vi "host.vi"() -> ()   [LabVIEW 2013]
uses:
  <vilib>/userdefined/High Color/nirio_resource_hc.ctl
  <instrlib>/niDCPower/nidcpower.llb/niDCPower Measurement Type.ctl
  <vilib>/FPGAPlugInAG/PXI-7953R/niLvFpga_Open_PXI-7953R.vi
  <vilib>/rvi/interface/common/dynamic/niFpgaDynamicAddResources.vi
  <vilib>/FPGAPlugInAG/Dynamic/niLvFpga_Reset_Dynamic.vi
  <vilib>/FPGAPlugInAG/Dynamic/niLvFpga_Run_Dynamic.vi
  <vilib>/rvi/interface/common/niFpgaWaitOnOcc.vi
  <vilib>/Utility/error.llb/Error Cluster From Error Code.vi
  <vilib>/rvi/errors/niLvFpgaAdjustHostInterfaceError.vi
  <vilib>/FPGAPlugInAG/Dynamic/niLvFpga_Close_Dynamic.vi
  <vilib>/rvi/interface/nirviOpenFPGA/nirviOpenFPGA.xnode
  FPGA Bitfiles/matrix_FPGATarget_Matrixtarget_8M6uhoGy8lc.lvbitx
  <vilib>/rvi/interface/nirviMethod/nirviMethod.xnode
  <vilib>/rvi/interface/nirviReadWriteControl/nirviReadWriteControl.xnode
  <vilib>/rvi/interface/nirviCloseFPGA/nirviCloseFPGA.xnode
  <vilib>/FPGAPlugInAG/Dynamic/niLvFpga_ReadFifo_Dynamic.vi
  <vilib>/rvi/errors/niLvFpgaMergeErrorWithErrorCode.vi
  <vilib>/rvi/interface/Simulation/niFpgaSimulationCallBeginRW.vi
  <vilib>/vision/NI_Vision_Development_Module.lvlib
  NiFpgaLv.dll
panel:
  in  "Мертвое время. мс":u32=200
  out "VAA_current, mA":dbl(graph)=0.09647506155015279
  out "VDDIO_current, mA":dbl(graph)=0.0007908422810211043
  out "VDD_current, mA":dbl(graph)=0.0007386855135800563
  in  "DELAY_i2c":u32=12
  out "Сумма сбоев":i32
  in  "Сброс Регистров":bool=TRUE
  out "Glitch Report":string
  in  "SEAL":bool
  in  "GLITCH":path=path "C:/TIM/Project/Matrix/Logs/Control/GLITCH"
  out "GLITCH_log file":refnum<file>
  in  "Index - Registers Page 2":u16[](array[numeric])=[2, 3, 4, 9, 10, 11, 12, 13, 14, 15, 16, 17, 65535, 65535, 65535, 21, 22, 23, 24, 25, 26, 27, 28, 29, 30, 31, 32, 33, 34, 35, 36, 38, 39, 40, 41, 42, 43, 44, 45, 46, 47, 65535, 65535, 65535, 51, 54, 55, 56, 57, 58, 59, 60, 61, 62, 65535, 70, 65535, 65535, 65535, 65535, 87, 88, 89, 90, 65535, 92, 93, 94, 95, 96, 65535, 65535, 65535, 100, 101, 103, 104, 130, 131, 132, 133, 134, 135, 136, 137, 138, 139, 140, 141, 142, 143, 144, 145, 146, 147, 148, 149, 150, 152, 153, 156, 180, 198, 200, 203, 204, 205, 206, 207, 208, 209, 210, 211, 212, 213, 239, 65535, 242, 65535, 244, 246, 247, 248, 249, 250, 251, 252, 253, 254, 255, 65535, 65535, 65535, 65535, 65535, 65535, 65535, 65535, 65534, 65535, 65535, 65531, 241, 242, 243, 244, 245, 246, 247, 248, 249, 250, 251, 252, 253, 254, 255]
  in  "Registers Page 2":u16[](array[numeric])=[110, 10531, 1316, 146, 22, 8, 171, 147, 88, 77, 169, 160, 65535, 65535, 65535, 373, 22, 67, 12, 0, 21, 31, 22, 152, 76, 160, 51220, 32896, 55648, 55648, 32512, 32768, 32776, 61188, 36211, 208, 24608, 24608, 61600, 3146, 57120, 65535, 65535, 65535, 5230, 30736, 768, 1088, 1676, 1676, 1676, 1676, 6105, 7423, 65535, 55552, 0, 65535, 65535, 65535, 537, 644, 537, 644, 2, 4620, 5394, 26684, 12296, 2, 32896, 65535, 65535, 23036, 0, 16400, 17, 1020, 769, 193, 929, 980, 983, 921, 1016, 28, 957, 987, 957, 1020, 990, 990, 990, 990, 31, 65, 867, 0, 255, 1, 57120, 32, 0, 0, 0, 0, 8608, 7835, 19018, 5773, 77, 0, 0, 520, 0, 8, 0, 0, 0, 110, 54, 13, 171, 136, 72, 87, 94, 122, 20543, 43136] format="%x"
  in  "current limit VDDIO":dbl=0.1 format="%#_13g"
  in  "voltage level VDDIO":dbl=2.5 format="%#_13g"
  in  "57":i16=57
  in  "91":i16=91
  in  "Index - Registers Page 1":u16[](array[numeric])=[5, 6, 8, 16, 17, 18, 27, 28, 30, 37, 52, 53, 58, 59, 60, 71, 72, 76, 77, 78, 82, 83, 84, 85, 86, 87, 88, 104, 128, 129, 130, 131, 132, 133, 134, 135, 136, 137, 138, 139, 140, 141, 142, 143, 144, 145, 146, 147, 148, 149, 155, 157, 159, 160, 161, 162, 163, 164, 165, 166, 167, 168, 169, 170, 174, 175, 179, 180, 181, 182, 183, 184, 185, 186, 187, 188, 189, 190, 191, 192, 193, 194, 195, 196, 200, 220, 221, 222, 223, 224, 225, 226, 227, 240]
  in  "Registers Page 1":u16[](array[numeric])=[3, 28686, 128, 61437, 64831, 16367, 0, 0, 512, 5, 16, 61456, 768, 1066, 1024, 24, 0, 0, 0, 10, 0, 7700, 17966, 34666, 47008, 57548, 0, 17, 7, 56588, 62696, 1276, 57868, 63212, 764, 56588, 62696, 250, 34866, 56754, 63466, 2, 47646, 60627, 63473, 255, 48926, 61142, 63474, 3, 512, 9390, 0, 1280, 1280, 0, 1024, 1024, 0, 1280, 640, 0, 1024, 512, 1284, 16, 2, 32, 257, 4363, 15399, 4362, 12834, 5643, 12836, 9228, 24124, 127, 8200, 20023, 100, 8463, 19250, 100, 0, 7700, 17966, 34666, 47008, 57548, 0, 28672, 45091, 0] format="%x"
  out "Glitch Registers":string
  out "glitch_num":i32
  out "Data_Read":u16 format="%x"
  in  "Index - Registers Page 0":u16[](array[numeric])=[0, 1, 2, 3, 4, 5, 6, 7, 8, 65535, 10, 11, 12, 13, 31, 32, 33, 34, 35, 36, 65535, 65535, 65535, 65535, 65535, 48, 49, 50, 51, 52, 54, 55, 65535, 60, 61, 65535, 63, 64, 65535, 66, 89, 90, 95, 96, 65535, 65535, 65535, 65535, 101, 112, 113, 114, 115, 116, 117, 118, 119, 120, 121, 122, 123, 124, 125, 126, 128, 129, 130, 131, 132, 133, 134, 135, 200, 240, 245, 246, 247, 248, 65535, 250, 251, 252, 253, 255, 65535]
  in  "Registers Page 0":u16[](array[numeric])=[5178, 12, 30, 1024, 487, 388, 42, 190, 17, 537, 17, 0, 0, 8, 0, 768, 1036, 297, 1544, 32875, 32, 32, 32, 32, 32, 1066, 7168, 0, 841, 49177, 61680, 0, 33, 6688, 8222, 8224, 8224, 8220, 215, 1911, 12, 49167, 8989, 128, 0, 0, 0, 0, 0, 31498, 31498, 6414, 6159, 22322, 22068, 29493, 12306, 30978, 29958, 30474, 30729, 32006, 12560, 126, 127, 127, 22282, 22539, 18188, 18446, 23298, 92, 0, 0, 2047, 2047, 0, 0, 124, 0, 0, 0, 0, 5178] format="%x"
  out "number":u64 format="%b"
  in  "WRITE\nSEL_LOG":bool=TRUE caption="SEL"
  out "SEL_log file":refnum<file>
  out "IS_SEL":bool
  in  "SIM_SEL":bool
  in  "VDDIO_limit, mA":dbl=20.0 format="%#_13g"
  in  "VAA_limit, mA":dbl=30.0 format="%#_13g"
  out "selNumVAA":i32 caption="selNum"
  out "selNumVDDIO":i32=3 caption="selNum"
  in  "voltage level VAA":dbl=2.8 format="%#_13g"
  in  "voltage level VDD":dbl=2.8 format="%#_13g"
  in  "current limit VAA":dbl=0.10000000000000009 format="%#_13g"
  in  "current limit VDD":dbl=0.1 format="%#_13g"
  in  "SEL":path=path "C:/TIM/Project/Matrix/Logs/Control/SEL"
  out "Температура":string="25"
  out "Номер образца":string="1"
  out "VDDIO_Current, mA":dbl=0.0007908422810211043 caption="mA" format="%_2g"
  out "VDDIO_Voltage, V":dbl=0.47498898751465163 caption="V" format="%_3g"
  out "VAA_Current, mA":dbl=0.09647506155015279 caption="mA" format="%_2g"
  out "VAA_Voltage, V":dbl=-0.00011092611436048789 caption="V" format="%_3g"
  in  "VAA - VAAPIX":refnum<k15>="PXI2Slot2"
  in  "SEL_time":u32=100
  out "Read_Low":u8 format="%x"
  out "Read_Up":u8 format="%x"
  out "TIRISTOR":bool
  in  "/RESET":bool=TRUE
  in  "DataLow":u8 format="%x"
  in  "Reg":u8=2 format="%x"
  in  "DataUp":u8 format="%x"
  in  "Device":u8=186 format="%x"
  in  "VDD_limit, mA":dbl=5.0 format="%#_13g"
  out "selNumVDD":i32 caption="selNum"
  out "Ready":bool
  in  "output enabled":bool
  out "VDD_Current, mA":dbl=0.0007386855135800563 caption="mA" format="%_2g"
  out "VDD_Voltage, V":dbl=0.00010885282841533817 caption="V" format="%_3g"
  in  "VDDIO - VDD":refnum<k15>="PXI2Slot3"
  in  "Comand":T1(ring)=enum."RGB565"
  in  "Height_pix":i32=250
  in  "Width_pix":i32=250
  in  "55":i16=55
  in  "73":i16=73
  in  "75":i16=75
  in  "56":i16=56
  in  "55":i16=55
  in  "Comand":bool
  out "ACK":u8 format="%b"
  out "String_counter":i16=250
  in  "String_number":i16=250
  in  "I2C_Request":bool
  in  "FALSE_LV":bool
  in  "FALSE_PIXCLK":bool
  in  "TRUE_FV":bool=TRUE
  in  "1_EXTCLK_divider":i16=3
  out "Image":T2(plugin-control)
  in  "0_WE divider":i32
  in  "50_Rise/Fall divider":i32=50
  in  "72":i16=72
  in  "18":i16=18
  in  "36":i16=36
  in  "54":i16=54
  in  "71":i16=71
  in  "17":i16=17
  in  "35":i16=35
  in  "53":i16=53
  in  "75_Stop":i16=75
  in  "100_Sclk_divider":i32=100
  in  "Read1":u8=255 format="%x"
  in  "Read2":u8=255 format="%x"
  in  "I2C_Write":bool=TRUE
  in  "stop":bool
  out "ArrayUp":u64=1408
  out "ArrayLow":u64=35465957116110822
  in  "resource name":T3="PXI2Slot6" caption="RIO Device"
  out "Сколько вначале":u32=125000
  out "Data":u8[](array[numeric])
  # "YCbCr mode"
  # "RGB565"
  # "LOGI"
  # "VDD"
  # "VDDIO"
  # "VAA"
  # "I2C"
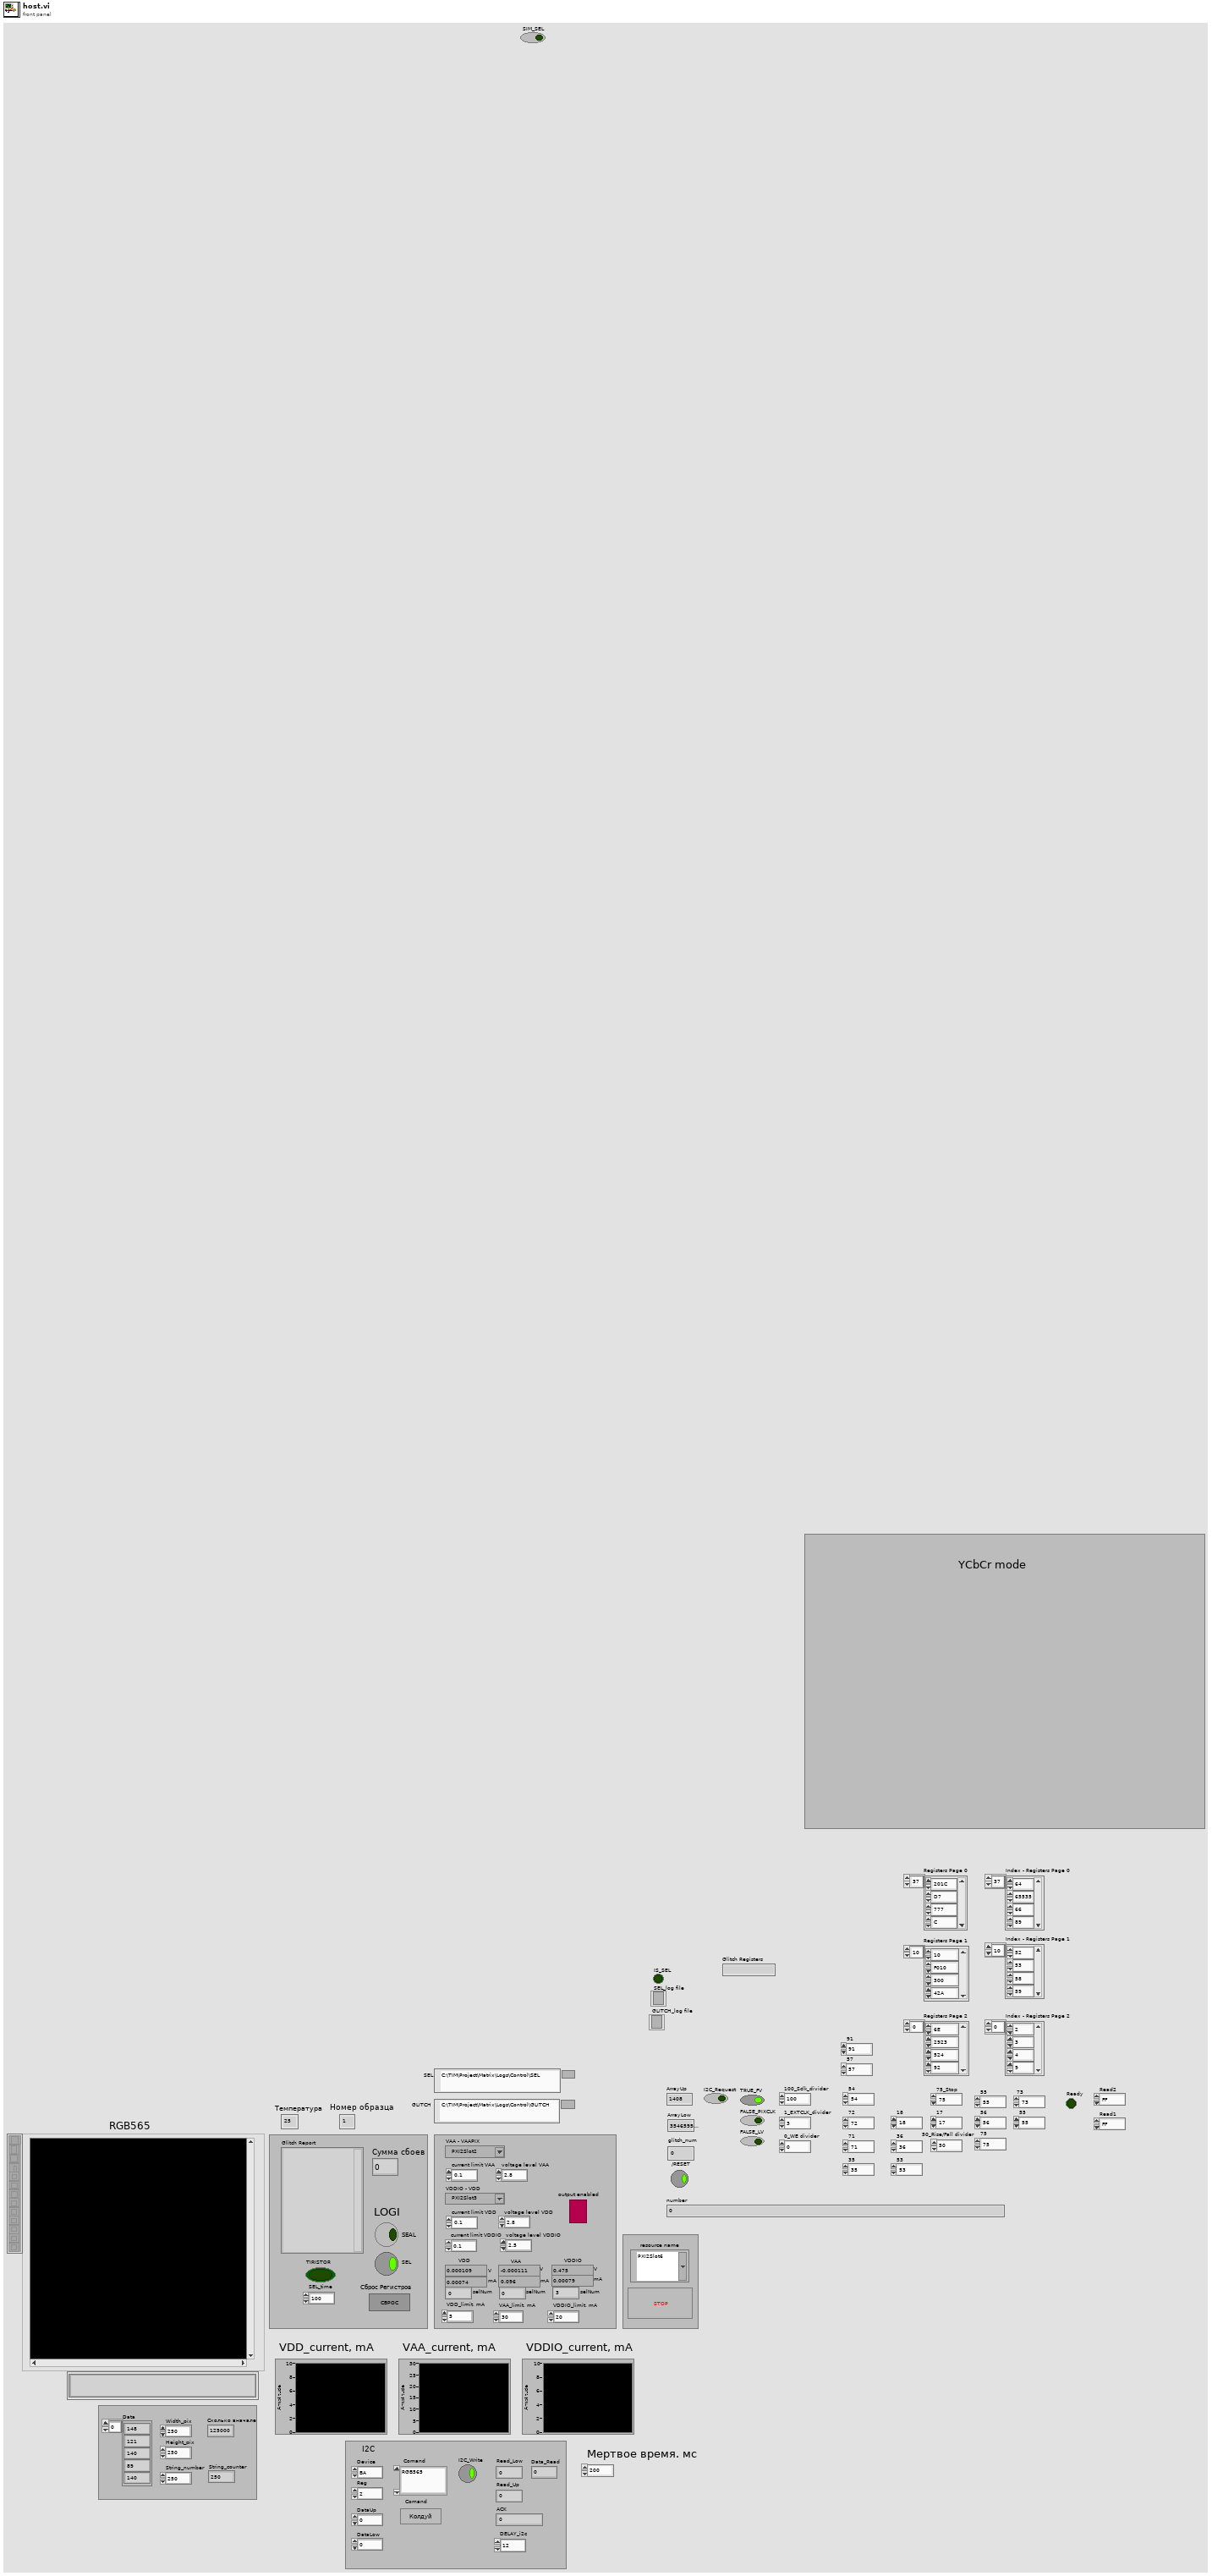
[diagram p1: front panel]
types:
  T1 = enum16{"check_registers", "From Controls", "250x250", "RGB565"}
  T2 = typedef "IMAQ Image.ctl" = refnum<image>
  T3 = typedef "nirio_resource_hc.ctl" = tag
  T4 = enum16{"open", "replace", "create", "open or create", "replace or create", "replace or create with confirmation"}
  T5 = typedef "niDCPower Measurement Type.ctl" = i32
  T6 = typedef "Image Type" = u32
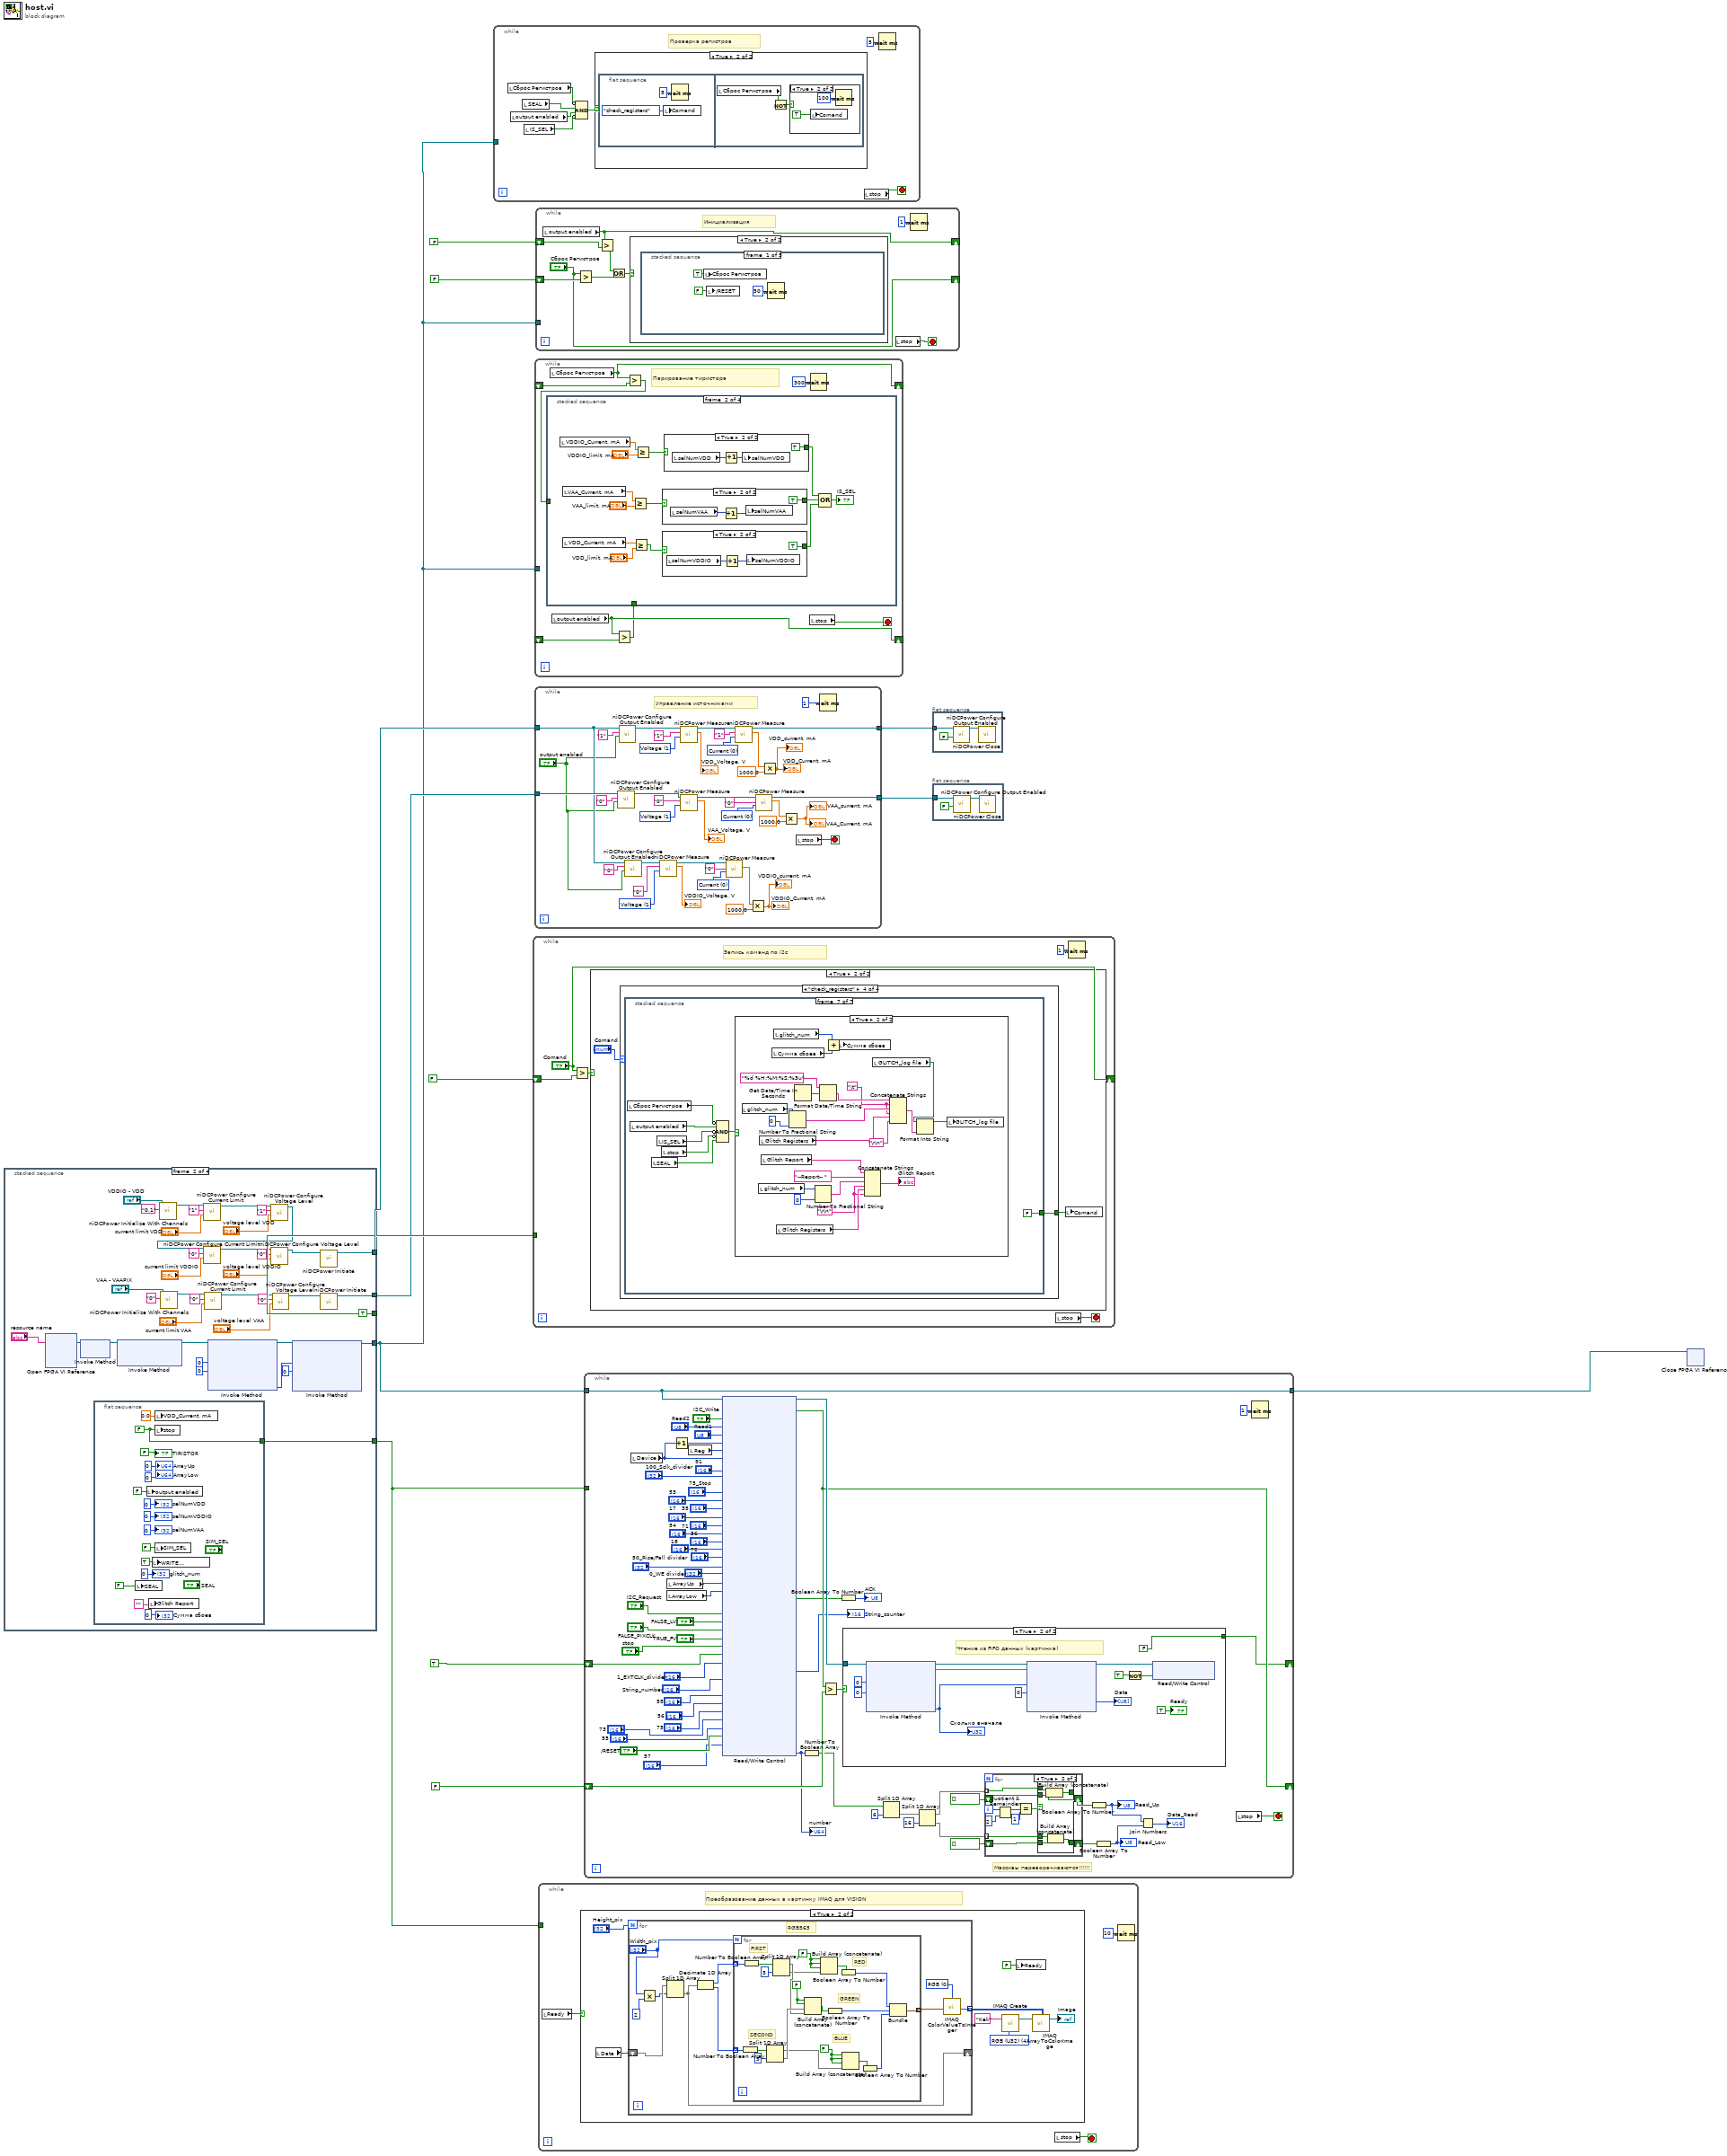
[diagram p0: block diagram]
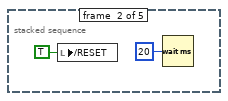
[diagram p3: hidden frame]
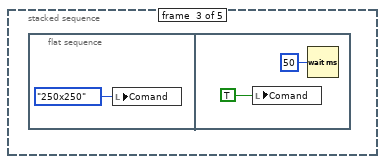
[diagram p4: hidden frame]
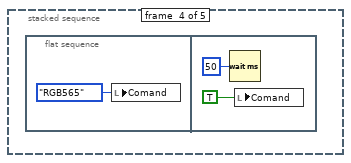
[diagram p5: hidden frame]
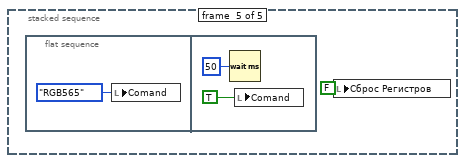
[diagram p6: hidden frame]
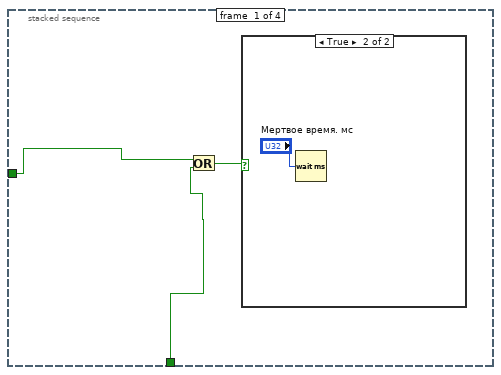
[diagram p10: hidden frame]
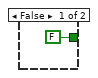
[diagram p12: hidden frame]
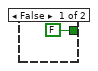
[diagram p13: hidden frame]
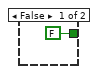
[diagram p14: hidden frame]
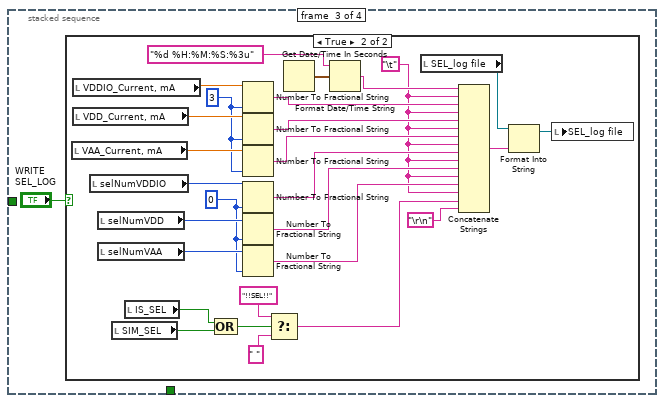
[diagram p15: hidden frame]
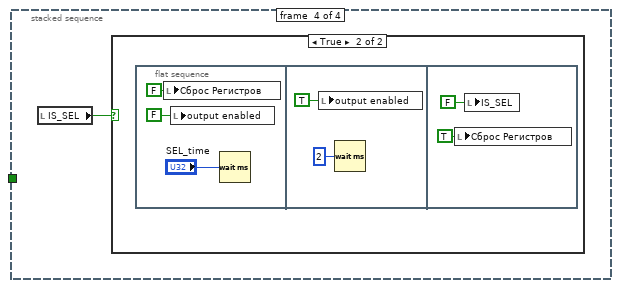
[diagram p17: hidden frame]
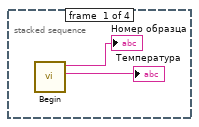
[diagram p19: hidden frame]
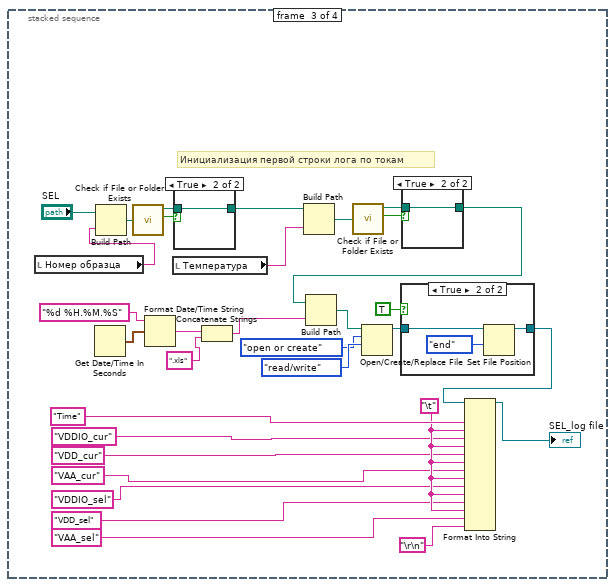
[diagram p20: hidden frame]
diagram:
  n1 = stacked-sequence {
    tunnel: [_ w53 _ _] -> w3
    tunnel: [_ w35 _ _] -> w6
    tunnel: [_ w34 _ _] -> w8
    tunnel: [_ TRUE _ _] -> w7
    tunnel: [_ w23 _ _] -> w5
    frame #0 {
      n2 = call "Begin.vi"() -> ("Температура 2"=→"Температура":string, "Номер образца 2"=→"Номер образца":string)  [unwired: 10 in]
    }
    frame #1 {
      n3 = xnode "Open FPGA VI Reference"("resource name"="resource name") -> ("FPGA VI Reference Out"=w44:refnum<k20>)  [unwired: 1 in, 1 out]
      n4 = xnode "Invoke Method"("FPGA VI Reference In"=w44) -> ("FPGA VI Reference Out"=w43:refnum<k20>)  [unwired: 1 in, 1 out]
      n5 = flat-sequence {
        tunnel: [w68] -> w35
        frame #0 {
          w68 = FALSE ("СТОП ПЛИС")
          n6 = local write "SEAL"(FALSE ("REGISTERS")) -> ()
          n7 = local write "output enabled"(FALSE ("output enabled")) -> ()
          n8 = local write "Glitch Report"("") -> ()
          n9 = local write "WRITE\nSEL_LOG"(TRUE ("WRITE\nSEL_LOG")) -> ()
          n10 = local write "VDD_Current, mA"(0.0 ("Ch1_Current, mA")) -> ()
          n11 = local write "stop"(w68) -> ()
          n12 = local write "SIM_SEL"(FALSE ("SIM_SEL")) -> ()
          "ArrayLow" <- u64 0 ("ArrayLow")
          "ArrayUp" <- u64 0 ("ArrayUp")
          "selNumVDD" <- 0 ("Numeric")
          "TIRISTOR" <- FALSE ("TIRISTOR")
          "selNumVDDIO" <- 0 ("Numeric")
          "selNumVAA" <- 0 ("Numeric")
          "glitch_num" <- 0 ("glitch_num")
          "Сумма сбоев" <- 0 ("glitch_sum")
        }
      }
      n13 = xnode "Invoke Method"("FPGA VI Reference In"=w43) -> ("FPGA VI Reference Out"=w41:refnum<k20>)  [unwired: 2 in, 1 out]
      n14 = call <instrlib>:"niDCPower Initialize With Channels.vi"("channels"="0,1", "resource name"="VDDIO - VDD") -> ("instrument handle out"=w45:refnum<k15>)  [unwired: 8 in, 1 out]
      n15 = call <instrlib>:"niDCPower Initialize With Channels.vi"("channels"="0", "resource name"="VAA - VAAPIX") -> ("instrument handle out"=w24:refnum<k15>)  [unwired: 8 in, 1 out]
      n16 = call <instrlib>:"niDCPower Configure Current Limit.vi"("current limit"="current limit VDD", "channel name"="1", "instrument handle"=w45) -> ("instrument handle out"=w46:refnum<k15>)  [unwired: 7 in, 1 out]
      n17 = call <instrlib>:"niDCPower Configure Current Limit.vi"("current limit"="current limit VAA", "channel name"="0", "instrument handle"=w24) -> ("instrument handle out"=w25:refnum<k15>)  [unwired: 7 in, 1 out]
      n18 = xnode "Invoke Method"("FPGA VI Reference In"=w41, "Number of Elements"=u32 0, "Timeout (ms)"=0) -> ("FPGA VI Reference Out"=w39:refnum<k20>, "Elements Remaining"=w40:u32)  [unwired: 1 in, 2 out]
      n19 = call <instrlib>:"niDCPower Configure Voltage Level.vi"("voltage level"="voltage level VDD", "channel name"="1", "instrument handle"=w46) -> ("instrument handle out"=w16:refnum<k15>)  [unwired: 7 in, 1 out]
      n20 = call <instrlib>:"niDCPower Configure Current Limit.vi"("current limit"="current limit VDDIO", "channel name"="0", "instrument handle"=w16) -> ("instrument handle out"=w22:refnum<k15>)  [unwired: 7 in, 1 out]
      n21 = call <instrlib>:"niDCPower Configure Voltage Level.vi"("voltage level"="voltage level VDDIO", "channel name"="0", "instrument handle"=w22) -> ("instrument handle out"=w17:refnum<k15>)  [unwired: 7 in, 1 out]
      n22 = call <instrlib>:"niDCPower Configure Voltage Level.vi"("voltage level"="voltage level VAA", "channel name"="0", "instrument handle"=w25) -> ("instrument handle out"=w26:refnum<k15>)  [unwired: 7 in, 1 out]
      n23 = xnode "Invoke Method"("FPGA VI Reference In"=w39, "Number of Elements"=w40, "Timeout (ms)"=0) -> ("FPGA VI Reference Out"=w53:refnum<k20>)  [unwired: 1 in, 3 out]
      n24 = call <instrlib>:"niDCPower Initiate.vi"("instrument handle"=w17) -> ("instrument handle out"=w34:refnum<k15>)  [unwired: 9 in, 1 out]
      n25 = call <instrlib>:"niDCPower Initiate.vi"("instrument handle"=w26) -> ("instrument handle out"=w23:refnum<k15>)  [unwired: 9 in, 1 out]
    }
    frame #2 {
      w77 = "\t"
      # "Инициализация первой строки лога по токам"
      n26 = local read "Номер образца"() -> (w88:string)
      n27 = Get Date/Time In Seconds() -> (seconds since 1Jan1904=w93:timestamp)
      n28 = Build Path(base path="SEL", name or relative path=w88) -> (appended path=w86:path)
      n29 = call <vilib>:"Check if File or Folder Exists.vi"("path"=w86) -> ("file or folder exists?"=w85:bool, "dup path"=w84:path)  [unwired: 8 in, 1 out]
      n30 = Format Date/Time String(time format string (%c)="%d %H.%M.%S", seconds (now)=w93) -> (date/time string=w95:string)  [unwired: 1 in]
      n31 = local read "Температура"() -> (w91:string)
      n32 = case shown="True" w85 {
        tunnel: w84 -> [w109 w110]
        tunnel: [w108 w110] -> w90
        frame False {
          n33 = Create Folder(path (use dialog)=w109) -> (created path=w108:path)  [unwired: 2 in, 2 out]
        }
        frame True {
        }
      }
      n34 = Concatenate Strings(w95, ".xls" ("string")) -> (w96:string)
      n35 = Build Path(base path=w90, name or relative path=w91) -> (appended path=w99:path)
      n36 = call <vilib>:"Check if File or Folder Exists.vi"("path"=w99) -> ("file or folder exists?"=w100:bool, "dup path"=w89:path)  [unwired: 8 in, 1 out]
      n37 = case shown="True" w100 {
        tunnel: w89 -> [w106 w107]
        tunnel: [w105 w107] -> w97
        frame False {
          n38 = Create Folder(path (use dialog)=w106) -> (created path=w105:path)  [unwired: 2 in, 2 out]
        }
        frame True {
        }
      }
      n39 = Build Path(base path=w97, name or relative path=w96) -> (appended path=w94:path)
      n40 = Open/Create/Replace File(file path (use dialog)=w94, operation (0:open)=T4."open or create", access (0:read/write)=enum16{"read/write", "read-only", "write-only"}."read/write") -> (refnum out=w92:refnum<file>)  [unwired: 3 in, 2 out]
      n41 = case shown="True" TRUE {
        tunnel: w92 -> [w101 w104]
        tunnel: [w101 w102] -> w98
        frame False {
        }
        frame True {
          n42 = Set File Position(refnum=w104, from (0:start)=enum16{"start", "end", "current"}."end") -> (refnum out=w102:refnum<file>)  [unwired: 2 in, 1 out]
        }
      }
      n43 = Format Into String(initial string=w98, "Time" ("input 1"), w77, "VDDIO_cur" ("input 1"), w77, "VDD_cur" ("input 1"), w77, "VAA_cur" ("input 1"), w77, "VDDIO_sel" ("input 1"), w77, "VDD_sel" ("input 1"), w77, "VAA_sel" ("input 1"), "\r\n") -> (resulting string=→"SEL_log file":refnum<file>)  [unwired: 2 in, 1 out]
    }
    frame #3 {
      w115 = "\t"
      # "Инициализация первой строки лога по сбоям"
      n44 = local read "Номер образца"() -> (w126:string)
      n45 = Get Date/Time In Seconds() -> (seconds since 1Jan1904=w131:timestamp)
      n46 = Build Path(base path="GLITCH", name or relative path=w126) -> (appended path=w124:path)
      n47 = call <vilib>:"Check if File or Folder Exists.vi"("path"=w124) -> ("file or folder exists?"=w123:bool, "dup path"=w122:path)  [unwired: 8 in, 1 out]
      n48 = Format Date/Time String(time format string (%c)="%d %H.%M.%S", seconds (now)=w131) -> (date/time string=w133:string)  [unwired: 1 in]
      n49 = local read "Температура"() -> (w129:string)
      n50 = case shown="True" w123 {
        tunnel: w122 -> [w147 w148]
        tunnel: [w146 w148] -> w128
        frame False {
          n51 = Create Folder(path (use dialog)=w147) -> (created path=w146:path)  [unwired: 2 in, 2 out]
        }
        frame True {
        }
      }
      n52 = Concatenate Strings(w133, ".xls" ("string")) -> (w134:string)
      n53 = Build Path(base path=w128, name or relative path=w129) -> (appended path=w137:path)
      n54 = call <vilib>:"Check if File or Folder Exists.vi"("path"=w137) -> ("file or folder exists?"=w138:bool, "dup path"=w127:path)  [unwired: 8 in, 1 out]
      n55 = case shown="True" w138 {
        tunnel: w127 -> [w144 w145]
        tunnel: [w143 w145] -> w135
        frame False {
          n56 = Create Folder(path (use dialog)=w144) -> (created path=w143:path)  [unwired: 2 in, 2 out]
        }
        frame True {
        }
      }
      n57 = Build Path(base path=w135, name or relative path=w134) -> (appended path=w132:path)
      n58 = Open/Create/Replace File(file path (use dialog)=w132, operation (0:open)=T4."open or create", access (0:read/write)=enum16{"read/write", "read-only", "write-only"}."read/write") -> (refnum out=w130:refnum<file>)  [unwired: 3 in, 2 out]
      n59 = case shown="True" TRUE {
        tunnel: w130 -> [w139 w142]
        tunnel: [w139 w140] -> w136
        frame False {
        }
        frame True {
          n60 = Set File Position(refnum=w142, from (0:start)=enum16{"start", "end", "current"}."end") -> (refnum out=w140:refnum<file>)  [unwired: 2 in, 1 out]
        }
      }
      n61 = Format Into String(initial string=w136, "Time" ("input 1"), w115, "Glitch Number" ("input 1"), w115, "Registers" ("input 1"), "\r\n") -> (resulting string=→"GLITCH_log file":refnum<file>)  [unwired: 2 in, 1 out]
    }
  }
  n62 = while {
    tunnel: w3 -> [_]
    stop <- w155 stop-if-true
    # "Проверка регистров"
    n63 = local read "Сброс Регистров"() -> (w149:bool)
    n64 = local read "output enabled"() -> (w153:bool)
    n65 = local read "SEAL"() -> (w152:bool)
    n66 = local read "IS_SEL"() -> (w151:bool)
    n67 = Compound Arithmetic op=AND(invert w149, w152, w153, invert w151) -> (w150:bool)
    n68 = case shown="True" w150 {
      frame False {
      }
      frame True {
        n69 = flat-sequence {
          frame #0 {
            n70 = local write "Comand"(T1."check_registers" ("Comand")) -> ()
            n71 = Wait (ms)(milliseconds to wait=u32 5) -> ()  [unwired: 1 out]
          }
          frame #1 {
            n72 = local read "Сброс Регистров"() -> (w159:bool)
            n73 = Not(x=w159) -> (.not. x?=w158:bool)
            n74 = case shown="True" w158 {
              frame False {
              }
              frame True {
                n75 = local write "Comand"(TRUE) -> ()
                n76 = Wait (ms)(milliseconds to wait=u32 100) -> ()  [unwired: 1 out]
              }
            }
          }
        }
      }
    }
    n77 = local read "stop"() -> (w155:bool)
    n78 = Wait (ms)(milliseconds to wait=u32 5) -> ()  [unwired: 1 out]
  }
  n79 = while {
    shift-right: ["Comand"] -> _
    shift-left: FALSE -> [w164]
    tunnel: w7 -> [_]
    stop <- w166 stop-if-true
    # "Запись команд по i2c"
    n80 = Greater?(x="Comand", y=w164) -> (0:w165:bool)
    n81 = case shown="True" w165 {
      frame False {
      }
      frame True {
        n82 = case shown="\"check_registers\"" "Comand" {
          tunnel: [w169 w195 w220 w232] -> w167
          frame "RGB565" {
            n83 = stacked-sequence {
              tunnel: [_ w181] -> w169
              frame #0 {
                n84 = flat-sequence {
                  frame #0 {
                    n85 = local write "I2C_Write"(TRUE ("I2C_Write")) -> ()
                    n86 = call "I2C_Write.vi"("DataLow"=u8 1 ("Device"), "DataUp"=u8 0 ("Device"), "Reg"=u8 240 ("Device"), "Device"=u8 186) -> ("ArrayLow"=w175:u64, "ArrayUp"=w174:u64)  [unwired: 6 in]
                    n87 = local write "ArrayUp"(w174) -> ()
                    n88 = local write "ArrayLow"(w175) -> ()
                  }
                  frame #1 {
                    n89 = local write "I2C_Request"(TRUE ("I2C_Request")) -> ()
                    n90 = Wait (ms)(milliseconds to wait=u32 20) -> ()  [unwired: 1 out]
                  }
                  frame #2 {
                    n91 = local write "I2C_Request"(FALSE ("I2C_Request")) -> ()
                    n92 = Wait (ms)(milliseconds to wait=u32 10) -> ()  [unwired: 1 out]
                  }
                }
              }
              frame #1 {
                n93 = flat-sequence {
                  tunnel: [FALSE ("RGB565")] -> w181
                  frame #0 {
                    n94 = local write "I2C_Write"(TRUE ("I2C_Write")) -> ()
                    n95 = call "I2C_Write.vi"("DataLow"=u8 0 ("Device"), "DataUp"=u8 3 ("Device"), "Reg"=u8 58 ("Device"), "Device"=u8 186) -> ("ArrayLow"=w187:u64, "ArrayUp"=w186:u64)  [unwired: 6 in]
                    n96 = local write "ArrayUp"(w186) -> ()
                    n97 = local write "ArrayLow"(w187) -> ()
                  }
                  frame #1 {
                    n98 = local write "I2C_Request"(TRUE ("I2C_Request")) -> ()
                    n99 = Wait (ms)(milliseconds to wait=u32 20) -> ()  [unwired: 1 out]
                  }
                  frame #2 {
                    n100 = local write "I2C_Request"(FALSE ("I2C_Request")) -> ()
                    n101 = Wait (ms)(milliseconds to wait=u32 10) -> ()  [unwired: 1 out]
                  }
                }
              }
            }
          }
          frame "250x250" {
            w194 = 250 ("Height_pix")
            n102 = stacked-sequence {
              tunnel: [_ w207] -> w195
              frame #0 {
                n103 = flat-sequence {
                  frame #0 {
                    n104 = local write "I2C_Write"(TRUE ("I2C_Write")) -> ()
                    n105 = call "I2C_Write.vi"("DataLow"=u8 0 ("Device"), "DataUp"=u8 0 ("Device"), "Reg"=u8 240 ("Device"), "Device"=u8 186) -> ("ArrayLow"=w201:u64, "ArrayUp"=w200:u64)  [unwired: 6 in]
                    n106 = local write "ArrayUp"(w200) -> ()
                    n107 = local write "ArrayLow"(w201) -> ()
                  }
                  frame #1 {
                    n108 = local write "I2C_Request"(TRUE ("I2C_Request")) -> ()
                    n109 = Wait (ms)(milliseconds to wait=u32 10) -> ()  [unwired: 1 out]
                  }
                  frame #2 {
                    n110 = local write "I2C_Request"(FALSE ("I2C_Request")) -> ()
                    n111 = Wait (ms)(milliseconds to wait=u32 10) -> ()  [unwired: 1 out]
                  }
                }
              }
              frame #1 {
                n112 = flat-sequence {
                  tunnel: [FALSE ("RGB565")] -> w207
                  frame #0 {
                    n113 = local write "I2C_Write"(TRUE ("I2C_Write")) -> ()
                    n114 = call "I2C_Write.vi"("DataLow"=u8 231 ("Device"), "DataUp"=u8 1 ("Device"), "Reg"=u8 4 ("Device"), "Device"=u8 186) -> ("ArrayLow"=w209:u64, "ArrayUp"=w208:u64)  [unwired: 6 in]
                    n115 = local write "ArrayUp"(w208) -> ()
                    n116 = local write "ArrayLow"(w209) -> ()
                  }
                  frame #1 {
                    n117 = local write "I2C_Request"(TRUE ("I2C_Request")) -> ()
                    n118 = Wait (ms)(milliseconds to wait=u32 10) -> ()  [unwired: 1 out]
                  }
                  frame #2 {
                    n119 = local write "I2C_Request"(FALSE ("I2C_Request")) -> ()
                    n120 = Wait (ms)(milliseconds to wait=u32 10) -> ()  [unwired: 1 out]
                  }
                }
              }
            }
            n121 = local write "String_number"(w194) -> ()
            n122 = local write "Width_pix"(w194) -> ()
            n123 = local write "Height_pix"(w194) -> ()
          }
          frame "From Controls" {
            n124 = flat-sequence {
              tunnel: [FALSE] -> w220
              frame #0 {
                n125 = call "I2C_Write.vi"("DataLow"="DataLow", "DataUp"="DataUp", "Reg"="Reg", "Device"="Device") -> ("ArrayLow"=w222:u64, "ArrayUp"=w221:u64)  [unwired: 6 in]
                n126 = local write "ArrayUp"(w221) -> ()
                n127 = local write "ArrayLow"(w222) -> ()
              }
              frame #1 {
                n128 = local write "I2C_Request"(TRUE ("I2C_Request")) -> ()
                n129 = Wait (ms)(milliseconds to wait=u32 20) -> ()  [unwired: 1 out]
              }
              frame #2 {
                n130 = local write "I2C_Request"(FALSE ("I2C_Request")) -> ()
                n131 = Wait (ms)(milliseconds to wait=u32 1) -> ()  [unwired: 1 out]
              }
            }
          }
          frame "check_registers" {
            n132 = stacked-sequence {
              tunnel: [_ _ _ _ _ _ FALSE ("RGB565")] -> w232
              frame #0 {
                n133 = flat-sequence {
                  frame #0 {
                    n134 = local write "I2C_Write"(TRUE ("I2C_Write")) -> ()
                    n135 = call "I2C_Write.vi"("DataLow"=u8 0 ("Device"), "DataUp"=u8 0 ("Device"), "Reg"=u8 240 ("Device"), "Device"=u8 186) -> ("ArrayLow"=w238:u64, "ArrayUp"=w237:u64)  [unwired: 6 in]
                    n136 = local write "ArrayUp"(w237) -> ()
                    n137 = local write "ArrayLow"(w238) -> ()
                  }
                  frame #1 {
                    n138 = local write "I2C_Request"(TRUE ("I2C_Request")) -> ()
                    n139 = Wait (ms)(milliseconds to wait="DELAY_i2c") -> ()  [unwired: 1 out]
                  }
                  frame #2 {
                    n140 = local write "I2C_Request"(FALSE ("I2C_Request")) -> ()
                    n141 = Wait (ms)(milliseconds to wait=u32 2) -> ()  [unwired: 1 out]
                  }
                }
              }
              frame #1 {
                # "PAGE 0"
                n142 = local write "glitch_num"(0 ("glitch_num")) -> ()
                n143 = local write "I2C_Write"(FALSE ("I2C_Write")) -> ()
                n144 = while {
                  tunnel: "Index - Registers Page 0" -> [w264] mode=indexing
                  tunnel: "Registers Page 0" -> [w263] mode=indexing
                  shift-right: [w261] -> w246
                  shift-left: "" -> [w262]
                  i -> [w257]
                  stop <- w255 stop-if-true
                  n145 = stacked-sequence {
                    tunnel: w264 -> [w266 _ w270]
                    tunnel: w263 -> [_ _ w275]
                    tunnel: w262 -> [_ _ w279]
                    tunnel: [_ _ w278] -> w261
                    frame #0 {
                      n146 = local write "Device"(u8 186 ("Device")) -> ()
                      n147 = local write "Reg"(w266) -> ()
                      n148 = Wait (ms)(milliseconds to wait=u32 4) -> ()  [unwired: 1 out]
                    }
                    frame #1 {
                      n149 = local write "I2C_Request"(TRUE ("I2C_Request")) -> ()
                      n150 = local read "DELAY_i2c"() -> (w268:u32)
                      n151 = Wait (ms)(milliseconds to wait=w268) -> ()  [unwired: 1 out]
                    }
                    frame #2 {
                      n152 = local read "Data_Read"() -> (w277:u16)
                      n153 = local write "I2C_Request"(FALSE ("I2C_Request")) -> ()
                      n154 = Equal?(x=w275, y=w277) -> (x = y?=w272:bool)
                      n155 = Equal?(x=w270, y=u16 65535) -> (x = y?=w274:bool)
                      n156 = Or(x=w272, y=w274) -> (x .or. y?=w271:bool)
                      n157 = case shown="False" w271 {
                        tunnel: w279 -> [w292 w295]
                        tunnel: [w291 w295] -> w278
                        tunnel: w270 -> [w289 _]
                        tunnel: w277 -> [w285 _]
                        tunnel: w275 -> [w281 _]
                        frame False {
                          n158 = local read "glitch_num"() -> (w294:i32)
                          n159 = Number To Hexadecimal String(2:w281) -> (0:w283:string)  [unwired: 1 in]
                          n160 = Number To Hexadecimal String(2:w285) -> (0:w287:string)  [unwired: 1 in]
                          n161 = Number To Decimal String(number=w289) -> (decimal integer string=w288:string)  [unwired: 1 in]
                          n162 = Increment(x=w294) -> (x+1=w293:i32)
                          n163 = call <vilib>:"Space Constant.vi"() -> ("String"=w282:string)
                          n164 = local write "glitch_num"(w293) -> ()
                          n165 = Concatenate Strings(w292, "p0#R" ("string"), w288, " rd ", w287, "  df  ", w283, w282) -> (w291:string)
                        }
                        frame True {
                        }
                      }
                      n166 = Wait (ms)(milliseconds to wait=u32 4) -> ()  [unwired: 1 out]
                    }
                  }
                  n167 = Wait (ms)(milliseconds to wait=u32 1) -> ()  [unwired: 1 out]
                  n168 = Greater Or Equal?(x=w257, y=82) -> (x >= y?=w258:bool)
                  n169 = local read "output enabled"() -> (w260:bool)
                  n170 = local read "SEAL"() -> (w252:bool)
                  n171 = local read "IS_SEL"() -> (w254:bool)
                  n172 = local read "stop"() -> (w253:bool)
                  n173 = Not(x=w260) -> (.not. x?=w259:bool)
                  n174 = Not(x=w252) -> (.not. x?=w251:bool)
                  n175 = Compound Arithmetic op=OR(w258, w259, w254, w253, w251) -> (w255:bool)
                }
                "Glitch Registers" <- w246
              }
              frame #2 {
                n176 = flat-sequence {
                  frame #0 {
                    n177 = local write "I2C_Write"(TRUE ("I2C_Write")) -> ()
                    n178 = call "I2C_Write.vi"("DataLow"=u8 1 ("Device"), "DataUp"=u8 0 ("Device"), "Reg"=u8 240 ("Device"), "Device"=u8 186) -> ("ArrayLow"=w301:u64, "ArrayUp"=w300:u64)  [unwired: 6 in]
                    n179 = local write "ArrayUp"(w300) -> ()
                    n180 = local write "ArrayLow"(w301) -> ()
                  }
                  frame #1 {
                    n181 = local read "DELAY_i2c"() -> (w303:u32)
                    n182 = local write "I2C_Request"(TRUE ("I2C_Request")) -> ()
                    n183 = Wait (ms)(milliseconds to wait=w303) -> ()  [unwired: 1 out]
                  }
                  frame #2 {
                    n184 = local write "I2C_Request"(FALSE ("I2C_Request")) -> ()
                    n185 = Wait (ms)(milliseconds to wait=u32 2) -> ()  [unwired: 1 out]
                  }
                }
              }
              frame #3 {
                # "PAGE 1"
                n186 = local read "Glitch Registers"() -> (w308:string)
                n187 = local write "I2C_Write"(FALSE ("I2C_Write")) -> ()
                n188 = while {
                  tunnel: "Index - Registers Page 1" -> [w323] mode=indexing
                  tunnel: "Registers Page 1" -> [w326] mode=indexing
                  shift-right: [w324] -> w307
                  shift-left: w308 -> [w325]
                  i -> [w317]
                  stop <- w319 stop-if-true
                  n189 = Wait (ms)(milliseconds to wait=u32 1) -> ()  [unwired: 1 out]
                  n190 = stacked-sequence {
                    tunnel: w323 -> [w328 _ w333]
                    tunnel: w326 -> [_ _ w337]
                    tunnel: w325 -> [_ _ w340]
                    tunnel: [_ _ w339] -> w324
                    frame #0 {
                      n191 = local write "Device"(u8 186 ("Device")) -> ()
                      n192 = local write "Reg"(w328) -> ()
                      n193 = Wait (ms)(milliseconds to wait=u32 2) -> ()  [unwired: 1 out]
                    }
                    frame #1 {
                      n194 = local write "I2C_Request"(TRUE ("I2C_Request")) -> ()
                      n195 = local read "DELAY_i2c"() -> (w330:u32)
                      n196 = Wait (ms)(milliseconds to wait=w330) -> ()  [unwired: 1 out]
                    }
                    frame #2 {
                      n197 = local read "Data_Read"() -> (w338:u16)
                      n198 = local write "I2C_Request"(FALSE ("I2C_Request")) -> ()
                      n199 = Equal?(x=w337, y=w338) -> (x = y?=w336:bool)
                      n200 = Equal?(x=w333, y=u16 65535) -> (x = y?=w335:bool)
                      n201 = Or(x=w336, y=w335) -> (x .or. y?=w334:bool)
                      n202 = case shown="False" w334 {
                        tunnel: w340 -> [w346 w357]
                        tunnel: [w347 w357] -> w339
                        tunnel: w333 -> [w345 _]
                        tunnel: w338 -> [w344 _]
                        tunnel: w337 -> [w343 _]
                        frame False {
                          n203 = local read "glitch_num"() -> (w356:i32)
                          n204 = Number To Decimal String(number=w345) -> (decimal integer string=w354:string)  [unwired: 1 in]
                          n205 = Number To Hexadecimal String(2:w344) -> (0:w353:string)  [unwired: 1 in]
                          n206 = Number To Hexadecimal String(2:w343) -> (0:w352:string)  [unwired: 1 in]
                          n207 = Increment(x=w356) -> (x+1=w355:i32)
                          n208 = call <vilib>:"Space Constant.vi"() -> ("String"=w348:string)
                          n209 = local write "glitch_num"(w355) -> ()
                          n210 = Concatenate Strings(w346, "p1#R" ("string"), w354, " rd ", w353, "  df  ", w352, w348) -> (w347:string)
                        }
                        frame True {
                        }
                      }
                      n211 = Wait (ms)(milliseconds to wait=u32 4) -> ()  [unwired: 1 out]
                    }
                  }
                  n212 = Greater Or Equal?(x=w317, y=75) -> (x >= y?=w318:bool)
                  n213 = local read "output enabled"() -> (w322:bool)
                  n214 = local read "SEAL"() -> (w315:bool)
                  n215 = local read "IS_SEL"() -> (w321:bool)
                  n216 = local read "stop"() -> (w314:bool)
                  n217 = Not(x=w322) -> (.not. x?=w320:bool)
                  n218 = Not(x=w315) -> (.not. x?=w313:bool)
                  n219 = Compound Arithmetic op=OR(w318, w320, w321, w314, w313) -> (w319:bool)
                }
                n220 = local write "Glitch Registers"(w307) -> ()
              }
              frame #4 {
                n221 = flat-sequence {
                  frame #0 {
                    n222 = local write "I2C_Write"(TRUE ("I2C_Write")) -> ()
                    n223 = call "I2C_Write.vi"("DataLow"=u8 2 ("Device"), "DataUp"=u8 0 ("Device"), "Reg"=u8 240 ("Device"), "Device"=u8 186) -> ("ArrayLow"=w363:u64, "ArrayUp"=w362:u64)  [unwired: 6 in]
                    n224 = local write "ArrayUp"(w362) -> ()
                    n225 = local write "ArrayLow"(w363) -> ()
                  }
                  frame #1 {
                    n226 = local read "DELAY_i2c"() -> (w365:u32)
                    n227 = local write "I2C_Request"(TRUE ("I2C_Request")) -> ()
                    n228 = Wait (ms)(milliseconds to wait=w365) -> ()  [unwired: 1 out]
                  }
                  frame #2 {
                    n229 = local write "I2C_Request"(FALSE ("I2C_Request")) -> ()
                    n230 = Wait (ms)(milliseconds to wait=u32 2) -> ()  [unwired: 1 out]
                  }
                }
              }
              frame #5 {
                # "PAGE 2"
                n231 = local read "Glitch Registers"() -> (w371:string)
                n232 = local write "I2C_Write"(FALSE ("I2C_Write")) -> ()
                n233 = while {
                  tunnel: "Index - Registers Page 2" -> [w386] mode=indexing
                  tunnel: "Registers Page 2" -> [w389] mode=indexing
                  shift-right: [w387] -> w370
                  shift-left: w371 -> [w388]
                  i -> [w380]
                  stop <- w379 stop-if-true
                  n234 = stacked-sequence {
                    tunnel: w386 -> [w391 _ w396]
                    tunnel: w389 -> [_ _ w400]
                    tunnel: w388 -> [_ _ w403]
                    tunnel: [_ _ w402] -> w387
                    frame #0 {
                      n235 = local write "Device"(u8 186 ("Device")) -> ()
                      n236 = local write "Reg"(w391) -> ()
                      n237 = Wait (ms)(milliseconds to wait=u32 2) -> ()  [unwired: 1 out]
                    }
                    frame #1 {
                      n238 = local write "I2C_Request"(TRUE ("I2C_Request")) -> ()
                      n239 = local read "DELAY_i2c"() -> (w393:u32)
                      n240 = Wait (ms)(milliseconds to wait=w393) -> ()  [unwired: 1 out]
                    }
                    frame #2 {
                      n241 = local read "Data_Read"() -> (w401:u16)
                      n242 = local write "I2C_Request"(FALSE ("I2C_Request")) -> ()
                      n243 = Equal?(x=w400, y=w401) -> (x = y?=w399:bool)
                      n244 = Equal?(x=w396, y=u16 65535) -> (x = y?=w398:bool)
                      n245 = Or(x=w399, y=w398) -> (x .or. y?=w397:bool)
                      n246 = case shown="False" w397 {
                        tunnel: w403 -> [w409 w420]
                        tunnel: [w410 w420] -> w402
                        tunnel: w396 -> [w408 _]
                        tunnel: w401 -> [w407 _]
                        tunnel: w400 -> [w406 _]
                        frame False {
                          n247 = local read "glitch_num"() -> (w419:i32)
                          n248 = Number To Decimal String(number=w408) -> (decimal integer string=w417:string)  [unwired: 1 in]
                          n249 = Number To Hexadecimal String(2:w407) -> (0:w416:string)  [unwired: 1 in]
                          n250 = Number To Hexadecimal String(2:w406) -> (0:w415:string)  [unwired: 1 in]
                          n251 = Increment(x=w419) -> (x+1=w418:i32)
                          n252 = call <vilib>:"Space Constant.vi"() -> ("String"=w411:string)
                          n253 = local write "glitch_num"(w418) -> ()
                          n254 = Concatenate Strings(w409, "p2#R" ("string"), w417, " rd ", w416, "  df  ", w415, w411) -> (w410:string)
                        }
                        frame True {
                        }
                      }
                      n255 = Wait (ms)(milliseconds to wait=u32 4) -> ()  [unwired: 1 out]
                    }
                  }
                  n256 = Wait (ms)(milliseconds to wait=u32 1) -> ()  [unwired: 1 out]
                  n257 = Greater Or Equal?(x=w380, y=129) -> (x >= y?=w382:bool)
                  n258 = local read "output enabled"() -> (w385:bool)
                  n259 = local read "SEAL"() -> (w378:bool)
                  n260 = local read "IS_SEL"() -> (w384:bool)
                  n261 = local read "stop"() -> (w377:bool)
                  n262 = Not(x=w385) -> (.not. x?=w383:bool)
                  n263 = Not(x=w378) -> (.not. x?=w376:bool)
                  n264 = Compound Arithmetic op=OR(w382, w383, w384, w377, w376) -> (w379:bool)
                }
                n265 = local write "Glitch Registers"(w370) -> ()
                n266 = Wait (ms)(milliseconds to wait=u32 4) -> ()  [unwired: 1 out]
              }
              frame #6 {
                n267 = local read "Сброс Регистров"() -> (w421:bool)
                n268 = local read "output enabled"() -> (w423:bool)
                n269 = local read "SEAL"() -> (w422:bool)
                n270 = local read "IS_SEL"() -> (w425:bool)
                n271 = local read "stop"() -> (w424:bool)
                n272 = Compound Arithmetic op=AND(invert w421, w423, invert w425, invert w424, w422) -> (w426:bool)
                n273 = case shown="True" w426 {
                  frame False {
                  }
                  frame True {
                    w431 = "\r\n"
                    w441 = "\t"
                    n274 = local read "glitch_num"() -> (w443:i32)
                    n275 = local read "glitch_num"() -> (w437:i32)
                    n276 = local read "Glitch Registers"() -> (w439:string)
                    n277 = local read "Glitch Report"() -> (w432:string)
                    n278 = local read "Сумма сбоев"() -> (w429:i32)
                    n279 = local read "glitch_num"() -> (w430:i32)
                    n280 = local read "Glitch Registers"() -> (w434:string)
                    n281 = Number To Fractional String(number=w443, precision (6)=i16 0 ("width (-)")) -> (F-format string=w442:string)  [unwired: 2 in]
                    n282 = Get Date/Time In Seconds() -> (seconds since 1Jan1904=w448:timestamp)
                    n283 = Number To Fractional String(number=w437, precision (6)=i16 0 ("width (-)")) -> (F-format string=w435:string)  [unwired: 2 in]
                    n284 = Format Date/Time String(time format string (%c)="%d %H:%M:%S:%3u", seconds (now)=w448) -> (date/time string=w450:string)  [unwired: 1 in]
                    n285 = Add(x=w430, y=w429) -> (x+y=w428:i32)
                    n286 = local write "Сумма сбоев"(w428) -> ()
                    n287 = Concatenate Strings(w432, "--Report-- ", w435, w431, w434, w431) -> (→"Glitch Report":string)
                    n288 = local read "GLITCH_log file"() -> (w447:refnum<file>)
                    n289 = Concatenate Strings(w450, w441, w442, w441, w439, "\r\n") -> (w449:string)
                    n290 = Format Into String(initial string=w447, w449) -> (resulting string=w446:refnum<file>)  [unwired: 2 in, 1 out]
                    n291 = local write "GLITCH_log file"(w446) -> ()
                  }
                }
              }
            }
          }
        }
        n292 = local write "Comand"(w167) -> ()
      }
    }
    n293 = local read "stop"() -> (w166:bool)
    n294 = Wait (ms)(milliseconds to wait=u32 1) -> ()  [unwired: 1 out]
  }
  n295 = while {
    tunnel: w3 -> [_]
    shift-right: [w455] -> _
    shift-left: _ -> [w456]
    shift-right: [w452] -> _
    shift-left: _ -> [w453]
    stop <- w458 stop-if-true
    # "Парирование тиристора"
    n296 = local read "Сброс Регистров"() -> (w455:bool)
    n297 = local read "output enabled"() -> (w452:bool)
    n298 = Greater?(x=w452, y=w453) -> (0:w451:bool)
    n299 = Greater?(x=w455, y=w456) -> (0:w454:bool)
    n300 = stacked-sequence {
      tunnel: w454 -> [w459 _ _ _]
      tunnel: w451 -> [w460 _ _ _]
      frame #0 {
        n301 = Or(x=w459, y=w460) -> (x .or. y?=w461:bool)
        n302 = case shown="True" w461 {
          frame False {
          }
          frame True {
            n303 = Wait (ms)(milliseconds to wait="Мертвое время. мс") -> ()  [unwired: 1 out]
          }
        }
      }
      frame #1 {
        n304 = local read "VDDIO_Current, mA"() -> (w470:dbl)
        n305 = local read "VAA_Current, mA"() -> (w471:dbl)
        n306 = local read "VDD_Current, mA"() -> (w475:dbl)
        n307 = Greater Or Equal?(x=w471, y="VAA_limit, mA") -> (x >= y?=w467:bool)
        n308 = Greater Or Equal?(x=w475, y="VDD_limit, mA") -> (x >= y?=w465:bool)
        n309 = Greater Or Equal?(x=w470, y="VDDIO_limit, mA") -> (x >= y?=w469:bool)
        n310 = case shown="True" w467 {
          tunnel: [FALSE TRUE] -> w466
          frame False {
          }
          frame True {
            n311 = local read "selNumVAA"() -> (w483:i32)
            n312 = Increment(x=w483) -> (x+1=w482:i32)
            n313 = local write "selNumVAA"(w482) -> ()
          }
        }
        n314 = case shown="True" w465 {
          tunnel: [FALSE TRUE] -> w464
          frame False {
          }
          frame True {
            n315 = local read "selNumVDDIO"() -> (w479:i32)
            n316 = Increment(x=w479) -> (x+1=w478:i32)
            n317 = local write "selNumVDDIO"(w478) -> ()
          }
        }
        n318 = case shown="True" w469 {
          tunnel: [FALSE TRUE] -> w468
          frame False {
          }
          frame True {
            n319 = local read "selNumVDD"() -> (w487:i32)
            n320 = Increment(x=w487) -> (x+1=w486:i32)
            n321 = local write "selNumVDD"(w486) -> ()
          }
        }
        n322 = Compound Arithmetic op=OR(w468, w466, w464) -> (→"IS_SEL":bool)
      }
      frame #2 {
        n323 = case shown="True" "WRITE\nSEL_LOG" {
          frame False {
          }
          frame True {
            w495 = i16 0 ("width (-)")
            w494 = i16 3 ("width (-)")
            w492 = "\t"
            n324 = local read "VAA_Current, mA"() -> (w509:dbl)
            n325 = local read "VDDIO_Current, mA"() -> (w507:dbl)
            n326 = local read "VDD_Current, mA"() -> (w508:dbl)
            n327 = local read "selNumVDDIO"() -> (w510:i32)
            n328 = local read "selNumVDD"() -> (w511:i32)
            n329 = local read "selNumVAA"() -> (w512:i32)
            n330 = local read "SIM_SEL"() -> (w499:bool)
            n331 = local read "IS_SEL"() -> (w500:bool)
            n332 = Compound Arithmetic op=OR(w500, w499) -> (w516:bool)
            n333 = Number To Fractional String(number=w507, precision (6)=w494) -> (F-format string=w513:string)  [unwired: 2 in]
            n334 = Number To Fractional String(number=w508, precision (6)=w494) -> (F-format string=w514:string)  [unwired: 2 in]
            n335 = Number To Fractional String(number=w509, precision (6)=w494) -> (F-format string=w515:string)  [unwired: 2 in]
            n336 = Number To Fractional String(number=w510, precision (6)=w495) -> (F-format string=w503:string)  [unwired: 2 in]
            n337 = Number To Fractional String(number=w511, precision (6)=w495) -> (F-format string=w502:string)  [unwired: 2 in]
            n338 = Number To Fractional String(number=w512, precision (6)=w495) -> (F-format string=w501:string)  [unwired: 2 in]
            n339 = Select(t="!!SEL!!", s=w516, f=" ") -> (s? t:f=w498:string)
            n340 = Get Date/Time In Seconds() -> (seconds since 1Jan1904=w504:timestamp)
            n341 = Format Date/Time String(time format string (%c)="%d %H:%M:%S:%3u", seconds (now)=w504) -> (date/time string=w506:string)  [unwired: 1 in]
            n342 = local read "SEL_log file"() -> (w490:refnum<file>)
            n343 = Concatenate Strings(w506, w492, w513, w492, w514, w492, w515, w492, w503, w492, w502, w492, w501, w492, w498, "\r\n") -> (w505:string)
            n344 = Format Into String(initial string=w490, w505) -> (resulting string=w489:refnum<file>)  [unwired: 2 in, 1 out]
            n345 = local write "SEL_log file"(w489) -> ()
          }
        }
      }
      frame #3 {
        n346 = local read "IS_SEL"() -> (w517:bool)
        n347 = case shown="True" w517 {
          frame False {
          }
          frame True {
            n348 = flat-sequence {
              frame #0 {
                n349 = local write "Сброс Регистров"(FALSE ("INIT_REGISTERS")) -> ()
                n350 = local write "output enabled"(FALSE ("output enabled")) -> ()
                n351 = Wait (ms)(milliseconds to wait="SEL_time") -> ()  [unwired: 1 out]
              }
              frame #1 {
                n352 = local write "output enabled"(TRUE ("output enabled")) -> ()
                n353 = Wait (ms)(milliseconds to wait=u32 2) -> ()  [unwired: 1 out]
              }
              frame #2 {
                n354 = local write "Сброс Регистров"(TRUE ("INIT_REGISTERS")) -> ()
                n355 = local write "IS_SEL"(FALSE ("IS_SEL")) -> ()
              }
            }
          }
        }
      }
    }
    n356 = local read "stop"() -> (w458:bool)
    n357 = Wait (ms)(milliseconds to wait=u32 300) -> ()  [unwired: 1 out]
  }
  n358 = while {
    tunnel: w8 -> [w527]
    tunnel: [w525] -> w10
    tunnel: w5 -> [w552]
    tunnel: [w553] -> w4
    stop <- w564 stop-if-true
    w531 = T5 0 items=["Current", "Voltage"] ("measurement type")
    w532 = T5 1 items=["Current", "Voltage"] ("measurement type")
    w543 = T5 0 items=["Current", "Voltage"] ("measurement type")
    w545 = T5 1 items=["Current", "Voltage"] ("measurement type")
    w555 = T5 0 items=["Current", "Voltage"] ("measurement type")
    w556 = T5 1 items=["Current", "Voltage"] ("measurement type")
    # "Управление источниками"
    n359 = call <instrlib>:"niDCPower Configure Output Enabled.vi"("output enabled"="output enabled", "channel name"="0", "instrument handle"=w552) -> ("instrument handle out"=w563:refnum<k15>)  [unwired: 7 in, 1 out]
    n360 = call <instrlib>:"niDCPower Configure Output Enabled.vi"("output enabled"="output enabled", "channel name"="1", "instrument handle"=w527) -> ("instrument handle out"=w538:refnum<k15>)  [unwired: 7 in, 1 out]
    n361 = call <instrlib>:"niDCPower Configure Output Enabled.vi"("output enabled"="output enabled", "channel name"="0", "instrument handle"=w527) -> ("instrument handle out"=w541:refnum<k15>)  [unwired: 7 in, 1 out]
    n362 = call <instrlib>:"niDCPower Measure.vi"("measurement type"=w545, "channel name"="0", "instrument handle"=w541) -> ("measurement"=→"VDDIO_Voltage, V":dbl, "instrument handle out"=w540:refnum<k15>)  [unwired: 6 in, 1 out]
    n363 = call <instrlib>:"niDCPower Measure.vi"("measurement type"=w532, "channel name"="1", "instrument handle"=w538) -> ("measurement"=→"VDD_Voltage, V":dbl, "instrument handle out"=w536:refnum<k15>)  [unwired: 6 in, 1 out]
    n364 = call <instrlib>:"niDCPower Measure.vi"("measurement type"=w556, "channel name"="0", "instrument handle"=w563) -> ("measurement"=→"VAA_Voltage, V":dbl, "instrument handle out"=w561:refnum<k15>)  [unwired: 6 in, 1 out]
    n365 = call <instrlib>:"niDCPower Measure.vi"("measurement type"=w543, "channel name"="0", "instrument handle"=w540) -> ("measurement"=w539:dbl)  [unwired: 6 in, 2 out]
    n366 = call <instrlib>:"niDCPower Measure.vi"("measurement type"=w531, "channel name"="1", "instrument handle"=w536) -> ("measurement"=w529:dbl, "instrument handle out"=w525:refnum<k15>)  [unwired: 6 in, 1 out]
    n367 = Multiply(x=w539, y=1000.0) -> (x*y=→"VDDIO_Current, mA" →"VDDIO_current, mA":dbl)
    n368 = call <instrlib>:"niDCPower Measure.vi"("measurement type"=w555, "channel name"="0", "instrument handle"=w561) -> ("measurement"=w557:dbl, "instrument handle out"=w553:refnum<k15>)  [unwired: 6 in, 1 out]
    n369 = Multiply(x=w529, y=1000.0) -> (x*y=→"VDD_Current, mA" →"VDD_current, mA":dbl)
    n370 = Multiply(x=w557, y=1000.0) -> (x*y=→"VAA_Current, mA" →"VAA_current, mA":dbl)
    n371 = local read "stop"() -> (w564:bool)
    n372 = Wait (ms)(milliseconds to wait=u32 1) -> ()  [unwired: 1 out]
  }
  n373 = while {
    shift-right: ["Сброс Регистров"] -> _
    shift-left: FALSE -> [w572]
    tunnel: w3 -> [_]
    shift-right: [w566] -> _
    shift-left: FALSE ("output enabled") -> [w568]
    stop <- w573 stop-if-true
    # "Инициализация"
    n374 = local read "output enabled"() -> (w566:bool)
    n375 = Greater?(x="Сброс Регистров", y=w572) -> (0:w569:bool)
    n376 = Greater?(x=w566, y=w568) -> (0:w567:bool)
    n377 = Or(x=w567, y=w569) -> (x .or. y?=w570:bool)
    n378 = case shown="True" w570 {
      frame False {
      }
      frame True {
        n379 = stacked-sequence {
          frame #0 {
            n380 = local write "Сброс Регистров"(TRUE ("INIT_REGISTERS")) -> ()
            n381 = local write "/RESET"(FALSE ("RESET")) -> ()
            n382 = Wait (ms)(milliseconds to wait=u32 50) -> ()  [unwired: 1 out]
          }
          frame #1 {
            n383 = local write "/RESET"(TRUE ("RESET")) -> ()
            n384 = Wait (ms)(milliseconds to wait=u32 20) -> ()  [unwired: 1 out]
          }
          frame #2 {
            n385 = flat-sequence {
              frame #0 {
                n386 = local write "Comand"(T1."250x250" ("Comand")) -> ()
              }
              frame #1 {
                n387 = local write "Comand"(TRUE) -> ()
                n388 = Wait (ms)(milliseconds to wait=u32 50) -> ()  [unwired: 1 out]
              }
            }
          }
          frame #3 {
            n389 = flat-sequence {
              frame #0 {
                n390 = local write "Comand"(T1."RGB565" ("Comand")) -> ()
              }
              frame #1 {
                n391 = Wait (ms)(milliseconds to wait=u32 50) -> ()  [unwired: 1 out]
                n392 = local write "Comand"(TRUE) -> ()
              }
            }
          }
          frame #4 {
            n393 = flat-sequence {
              frame #0 {
                n394 = local write "Comand"(T1."RGB565" ("Comand")) -> ()
              }
              frame #1 {
                n395 = Wait (ms)(milliseconds to wait=u32 50) -> ()  [unwired: 1 out]
                n396 = local write "Comand"(TRUE) -> ()
              }
            }
            n397 = local write "Сброс Регистров"(FALSE) -> ()
          }
        }
      }
    }
    n398 = local read "stop"() -> (w573:bool)
    n399 = Wait (ms)(milliseconds to wait=u32 1) -> ()  [unwired: 1 out]
  }
  n400 = while {
    tunnel: w6 -> [_]
    stop <- w591 stop-if-true
    # "Преобразование данных в картинку IMAQ для VISION"
    n401 = local read "Ready"() -> (w589:bool)
    n402 = case shown="True" w589 {
      frame False {
      }
      frame True {
        w598 = T6 4 items=["Grayscale (U8)", "Grayscale (I16)", "Grayscale (SGL)", "Complex (CSG)", "RGB (U32)", "HSL (U32)", "RGB (U64)"] ("Image Type")
        n403 = local read "Data"() -> (w593:u8[])
        n404 = for {
          N: "Height_pix" -> [_]
          shift-right: [w605] -> _
          shift-left: w593 -> [w602]
          tunnel: [w603] -> w594 mode=indexing
          w607 = u16 0 items=["RGB", "HSL", "HSV", "HSI"] ("Color Mode")
          # "RGB565"
          n405 = Multiply(x="Width_pix", y=2) -> (x*y=w601:i32)
          n406 = Split 1D Array(array=w602, index=w601) -> (second subarray=w605:u8[])  [unwired: 1 out]
          n407 = Decimate 1D Array(w605) -> (w609:u8[], w608:u8[])
          n408 = for {
            N: "Width_pix" -> [_]
            tunnel: w609 -> [w628] mode=indexing
            tunnel: w608 -> [w629] mode=indexing
            tunnel: [w610] -> w604 mode=indexing
            w618 = FALSE
            w619 = FALSE
            w620 = FALSE
            # "BLUE"
            # "GREEN"
            # "RED"
            # "SECOND"
            # "FIRST"
            n409 = Number To Boolean Array(number=w629) -> (Boolean array=w624:bool[])
            n410 = Number To Boolean Array(number=w628) -> (Boolean array=w627:bool[])
            n411 = Split 1D Array(array=w624, index=5) -> (first subarray=w616:bool[], second subarray=w623:bool[])
            n412 = Split 1D Array(array=w627, index=3) -> (first subarray=w615:bool[], second subarray=w614:bool[])
            n413 = Build Array (concatenate)(w619, w619, w623, w615) -> (w622:bool[])
            n414 = Build Array (concatenate)(w620, w620, w620, w614) -> (w621:bool[])
            n415 = Boolean Array To Number(Boolean array=w622) -> (number=w612:u8)
            n416 = Boolean Array To Number(Boolean array=w621) -> (number=w611:u8)
            n417 = Build Array (concatenate)(w618, w618, w618, w616) -> (w617:bool[])
            n418 = Boolean Array To Number(Boolean array=w617) -> (number=w613:u8)
            n419 = Bundle(w611, w612, w613) -> (w610:cluster{u8, u8, u8})  [unwired: 1 in]
          }
          n420 = call "IMAQ ColorValueToInteger"("1D Color value array"=w604, "Color Mode"=w607) -> ("1D U32 array"=w603:u32[])  [unwired: 3 in, 3 out]
        }
        n421 = call "IMAQ Create"("Image Name"="Kek", "Image Type"=w598) -> ("New Image"=w597:T2)  [unwired: 3 in, 1 out]
        n422 = local write "Ready"(FALSE ("Ready")) -> ()
        n423 = call "IMAQ ArrayToColorImage"("Image Pixels (U32)"=w594, "Image"=w597) -> ("Image Out"=→"Image":T2)  [unwired: 3 in, 1 out]
      }
    }
    n424 = local read "stop"() -> (w591:bool)
    n425 = Wait (ms)(milliseconds to wait=u32 10) -> ()  [unwired: 1 out]
  }
  n426 = while {
    tunnel: w3 -> [w689]
    tunnel: [w689] -> w13
    shift-right: [w671] -> _
    shift-left: FALSE -> [w690]
    tunnel: w6 -> [_]
    shift-right: [w652] -> _
    shift-left: TRUE -> [w653]
    stop <- w651 stop-if-true
    # "Массивы переворачиваются!!!!!!"
    n427 = local read "Device"() -> (w648:u8)
    n428 = local read "ArrayLow"() -> (w665:u64)
    n429 = local read "ArrayUp"() -> (w664:u64)
    n430 = Increment(x=w648) -> (x+1=w647:u8)
    n431 = local read "Reg"() -> (w646:u8)
    n432 = xnode "Read/Write Control"("FPGA VI Reference In"=w689, "I2C_Write"="I2C_Write", "Read2"="Read2", "Read1"="Read1", "Device_Read"=w647, "Reg"=w646, "Device_Write"=w648, "91"="91", "100_Sclk_divider"="100_Sclk_divider", "75_Stop"="75_Stop", "53"="53", "35"="35", "17"="17", "71"="71", "54"="54", "36"="36", "18"="18", "72"="72", "50_Rise/Fall divider"="50_Rise/Fall divider", "0_WE divider"="0_WE divider", "DataUp"=w664, "DataLow"=w665, "I2C_Request"="I2C_Request", "FALSE_LV"="FALSE_LV", "FALSE_PIXCLK"="FALSE_PIXCLK", "TRUE_FV"="TRUE_FV", "Остановите"="stop", "Читай_Линию"=w653, "1_EXTCLK_divider"="1_EXTCLK_divider", "String_number"="String_number", "55"="55", "56"="56", "75"="75", "73"="73", "55"="55", "RESET"="/RESET", "57"="57") -> ("FPGA VI Reference Out"=w688:refnum<k20>, "Линия_готова_на_все"=w671:bool, "ACK"=w660:bool[], "String_counter"=→"String_counter":i16, "READ_Number"=w632:u64)  [unwired: 2 in, 3 out]
    "number" <- w632
    n433 = Number To Boolean Array(number=w632) -> (Boolean array=w633:bool[])
    n434 = Greater?(x=w671, y=w690) -> (0:w661:bool)
    n435 = Boolean Array To Number(Boolean array=w660) -> (number=→"ACK":u8)
    n436 = case shown="True" w661 {
      tunnel: w688 -> [_ w718]
      tunnel: [TRUE FALSE ("Читай_Линию")] -> w652
      frame False {
      }
      frame True {
        # "Чтение из FIFO данных (картинка)"
        n437 = xnode "Invoke Method"("FPGA VI Reference In"=w718, "Number of Elements"=u32 0, "Timeout (ms)"=0) -> ("FPGA VI Reference Out"=w723:refnum<k20>, "error out"=w722:errorcluster, "Elements Remaining"=w714:u32)  [unwired: 1 in, 1 out]
        "Сколько вначале" <- w714
        n438 = xnode "Invoke Method"("FPGA VI Reference In"=w723, "error in"=w722, "Number of Elements"=w714, "Timeout (ms)"=0) -> ("FPGA VI Reference Out"=w715:refnum<k20>, "Data"=→"Data":u8[])  [unwired: 2 out]
        n439 = Not(x=TRUE) -> (.not. x?=w716:bool)
        n440 = xnode "Read/Write Control"("FPGA VI Reference In"=w715, "Линия_ прочтена"=w716) -> ()  [unwired: 1 in, 2 out]
        "Ready" <- TRUE ("Ready")
      }
    }
    n441 = Split 1D Array(array=w633, index=6) -> (second subarray=w644:bool[])  [unwired: 1 out]
    n442 = Split 1D Array(array=w644, index=16) -> (first subarray=w642:bool[], second subarray=w640:bool[])
    n443 = for {
      tunnel: w642 -> [w701] mode=indexing
      shift-right: [w700] -> w641
      shift-left: bool[] [] -> [w699]
      tunnel: w640 -> [w693] mode=indexing
      shift-right: [w692] -> w639
      shift-left: bool[] [] -> [w691]
      i -> [w696]
      n444 = Quotient & Remainder(x=w696, y=2) -> (x-y*floor(x/y)=w698:i32)  [unwired: 1 out]
      n445 = Equal?(x=w698, y=1) -> (x = y?=w697:bool)
      n446 = case shown="True" w697 {
        tunnel: w701 -> [_ w709]
        tunnel: [w703 w708] -> w700
        tunnel: w699 -> [w703 w707]
        tunnel: w693 -> [_ w706]
        tunnel: [w702 w705] -> w692
        tunnel: w691 -> [w702 w704]
        frame False {
        }
        frame True {
          n447 = Build Array (concatenate)(w709, w707) -> (w708:bool[])
          n448 = Build Array (concatenate)(w706, w704) -> (w705:bool[])
        }
      }
    }
    n449 = Boolean Array To Number(Boolean array=w641) -> (number=w631:u8)
    "Read_Up" <- w631
    n450 = Boolean Array To Number(Boolean array=w639) -> (number=w630:u8)
    "Read_Low" <- w630
    n451 = Join Numbers(hi=w631, lo=w630) -> ((hi.lo)=→"Data_Read":u16)
    n452 = local read "stop"() -> (w651:bool)
    n453 = Wait (ms)(milliseconds to wait=u32 1) -> ()  [unwired: 1 out]
  }
  n454 = flat-sequence {
    tunnel: w10 -> [w726]
    frame #0 {
      n455 = call <instrlib>:"niDCPower Configure Output Enabled.vi"("output enabled"=FALSE, "instrument handle"=w726) -> ("instrument handle out"=w724:refnum<k15>)  [unwired: 8 in, 1 out]
      n456 = call <instrlib>:"niDCPower Close.vi"("instrument handle"=w724) -> ()  [unwired: 10 in, 1 out]
    }
  }
  n457 = flat-sequence {
    tunnel: w4 -> [w729]
    frame #0 {
      n458 = call <instrlib>:"niDCPower Configure Output Enabled.vi"("output enabled"=FALSE, "instrument handle"=w729) -> ("instrument handle out"=w727:refnum<k15>)  [unwired: 8 in, 1 out]
      n459 = call <instrlib>:"niDCPower Close.vi"("instrument handle"=w727) -> ()  [unwired: 10 in, 1 out]
    }
  }
  n460 = xnode "Close FPGA VI Reference"("FPGA VI Reference In"=w13) -> ()  [unwired: 1 in, 1 out]
